vi "NotifyIcon - Get MenuItem.vi"(8 "error in":errorcluster, 10 "Context MenuItem":string="submenu/MenuItem", 11 "NotifyIcon reference in":refnum<k24>) -> (0 "error out":errorcluster, 1 "MenuItem reference":refnum<k24>, 3 "NotifyIcon reference out":refnum<k24>)   [LabVIEW 2009]
doc: "Returns a reference to a MenuItem specified by <b>Context MenuItem</b>\n\nTo reference a MenuItem in a sub-menu, use the following format:\nsubmenu/MenuItem"
uses:
  System.Windows.Forms
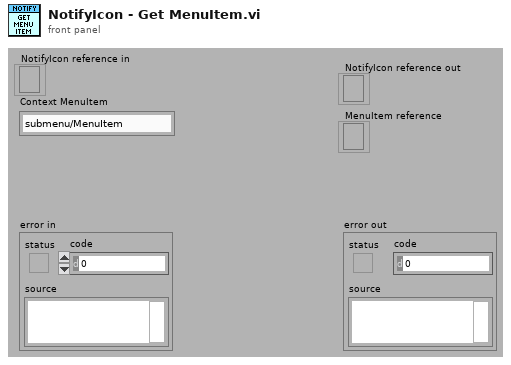
[diagram p1: front panel]
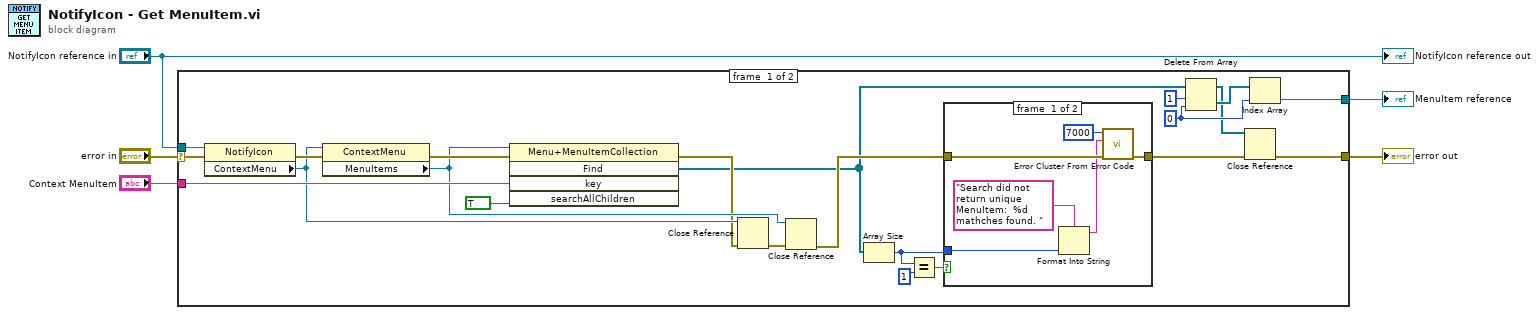
[diagram p0: block diagram]
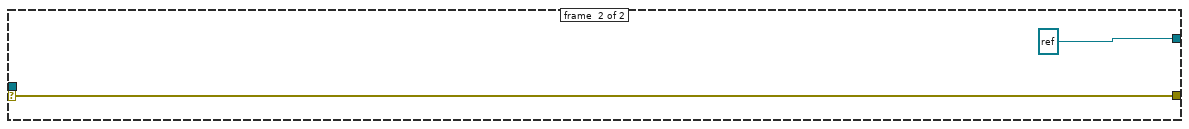
[diagram p3: hidden frame]
diagram:
  n1 = case shown="No Error" "error in" {
    selector: "error in" -> [w19 w36]
    tunnel: "NotifyIcon reference in" -> [w27 _]
    tunnel: "Context MenuItem" -> [w23 _]
    tunnel: [w11 w36] -> w3
    tunnel: [w13 refnum<k24> refnum] -> w2
    frame #0 {
      w9 = 0 ("index")
      n2 = property class="NotifyIcon"(reference=w27, error in=w19) -> (error out=w26:errorcluster, "ContextMenu"=w18:refnum<k24>)  [unwired: 1 out]
      n3 = property class="ContextMenu"(reference=w18, error in=w26) -> (error out=w25:errorcluster, "MenuItems"=w17:refnum<k24>)  [unwired: 1 out]
      n4 = invoke class="Menu+MenuItemCollection" method="Find"(reference=w17, error in=w25, "key"=w23, "searchAllChildren"=TRUE) -> (error out=w16:errorcluster, "Find"=w10:refnum<k24>[])  [unwired: 1 in, 3 out]
      n5 = Close Reference(reference=w18, error in (no error)=w16) -> (error out=w15:errorcluster)
      n6 = Close Reference(reference=w17, error in (no error)=w15) -> (error out=w14:errorcluster)
      n7 = Array Size(array=w10) -> (size(s)=w21:i32)
      n8 = Equal?(x=w21, y=1) -> (x = y?=w20:bool)
      n9 = case shown="False" w20 {
        tunnel: w14 -> [w32 w34]
        tunnel: [w33 w34] -> w12
        tunnel: w21 -> [w29 _]
        frame #0 {
          n10 = Format Into String(format string="Search did not return unique MenuItem:  %d mathches found. " ("error message (\"\")"), w29) -> (resulting string=w28:string)  [unwired: 2 in, 1 out]
          n11 = call <vilib>:"Error Cluster From Error Code.vi"("error in (no error)"=w32, "error message (\"\")"=w28, "error code (0)"=7000) -> ("error out"=w33:errorcluster)  [unwired: 6 in]
        }
        frame #1 {
        }
      }
      n12 = Delete From Array(array=w10, length=1, index=w9) -> (deleted portion=w7:refnum<k24>[], array with subset deleted=w6:refnum<k24>[])
      n13 = Close Reference(reference=w6, error in (no error)=w12) -> (error out=w11:errorcluster)
      n14 = Index Array(array=w7, index=w9) -> (element=w13:refnum<k24>)
    }
    frame #1 {
    }
  }
  "MenuItem reference" <- w2
  "error out" <- w3
  "NotifyIcon reference out" <- "NotifyIcon reference in"
